vi "Data Logging.old.vi"(8 "error in (no error)":errorcluster, 11 "stop?":bool) -> (0 "error out":errorcluster)   [LabVIEW 2011]
uses:
  <vilib>/Utility/sysdir.llb/System Directory Type.ctl
  <vilib>/Platform/TimedLoop/XDataNode/timing_clust.ctl
  <vilib>/Platform/TimedLoop/XDataNode/nitl_modes.ctl
  <vilib>/Platform/TimedLoop/XDataNode/wakeup.ctl
  <vilib>/Platform/TimedLoop/XDataNode/XDataNode.xnode
  <vilib>/Platform/TimedLoop/XDataNode/XDNodeRunTimeDep.lvlib
panel:
  out "Data Cluster":T1
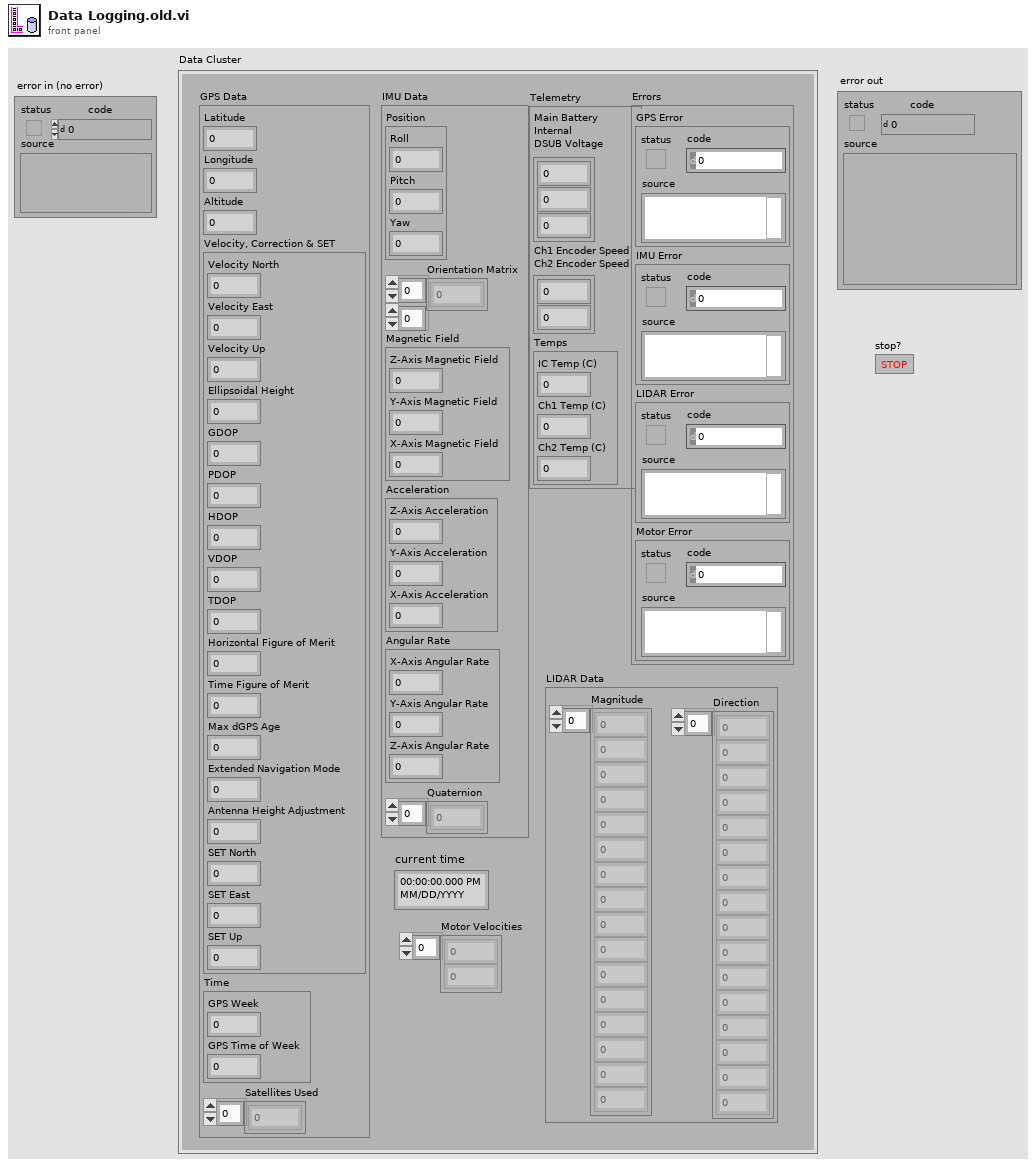
[diagram p1: front panel]
types:
  T1 = cluster{"GPS Data":cluster{"Latitude":dbl, "Longitude":dbl, "Altitude":dbl, "Velocity, Correction & SET":cluster{"Velocity North":dbl, "Velocity East":dbl, "Velocity Up":dbl, "Ellipsoidal Height":dbl, "GDOP":sgl, "PDOP":sgl, "HDOP":sgl, "VDOP":sgl, "TDOP":sgl, "Horizontal Figure of Merit":u8, "Time Figure of Merit":u8, "Max dGPS Age":sgl, "Extended Navigation Mode":u8, "Antenna Height Adjustment ":dbl, "SET North":i32, "SET East":i32, "SET Up":i32}, "Time":cluster{"GPS Week":u16, "GPS Time of Week":sgl}, "Satellites Used":i32[]}, "IMU Data":cluster{"Position":cluster{"Roll":dbl, "Pitch":dbl, "Yaw":dbl}, "Orientation Matrix":dbl[][], "Magnetic Field":cluster{"Z-Axis Magnetic Field":dbl, "Y-Axis Magnetic Field":dbl, "X-Axis Magnetic Field":dbl}, "Acceleration":cluster{"Z-Axis Acceleration":dbl, "Y-Axis Acceleration":dbl, "X-Axis Acceleration":dbl}, "Angular Rate":cluster{"X-Axis Angular Rate":dbl, "Y-Axis Angular Rate":dbl, "Z-Axis Angular Rate":dbl}, "Quaternion":dbl[]}, "Telemetry":cluster{"Main Battery\nInternal\nDSUB Voltage":cluster{sgl, sgl, sgl}, "Ch1 Encoder Speed\nCh2 Encoder Speed":cluster{i32, i32}, "Temps":cluster{"IC Temp (C)":i32, "Ch1 Temp (C)":i32, "Ch2 Temp (C)":i32}}, "Motor Velocities":dbl[], "Errors":cluster{"GPS Error ":errorcluster, "IMU Error":errorcluster, "LIDAR Error":errorcluster, "Motor Error":errorcluster}, "current time":timestamp, "LIDAR Data":cluster{"Magnitude":dbl[], "Direction":dbl[]}}
  T2 = enum16{"open", "replace", "create", "open or create", "replace or create", "replace or create with confirmation"}
  T3 = typedef "System Directory Type.ctl" = i32
  T4 = cluster{"GPS Error ":errorcluster, "IMU Error":errorcluster, "LIDAR Error":errorcluster, "Motor Error":errorcluster}
  T5 = typedef "XDNodeRunTimeDep.lvlib/timing_clust.ctl" = cluster{"Expected End [f-1]":u64, "Actual End [f-1]":u64, "Finished Late? [f-1]":bool, "Expected End [i-1]":u64, "Actual End [i-1]":u64, "Finished Late? [i-1]":bool, "Expected Start [i]":u64, "Actual Start [i]":u64, "Expected Start [f]":u64, "Actual Start [f]":u64, "Source Name":string, "Structure Name":string, "Period":i64, "Deadline":i64, "Offset":i64, "Start":i64, "Priority":i32, "Timeout":i32, "Mode":T6, "Wakeup Reason":T7, "Error":errorcluster, "Source Type":string, "Secondary Source Type":string, "Global End Time":u64, "Global Start Time":u64, "Frame Duration":u64, "Iteration Duration":u64, "Assigned CPU":i32, "I/O Scan Engine Mode":u32}
  T6 = typedef "XDNodeRunTimeDep.lvlib/nitl_modes.ctl" = enum32{"No Change", "Process missed periods, maintain original phase", "Discard missed periods, maintain original phase", "Process missed periods, ignore original phase", "Discard missed periods, ignore original phase"}
  T7 = typedef "XDNodeRunTimeDep.lvlib/wakeup.ctl" = enum32{"Normal", "Aborted", "Asynchronous wakeup", "Timing source error", "Timed loop error", "Timeout"}
  T8 = cluster{"Main Battery\nInternal\nDSUB Voltage":cluster{sgl, sgl, sgl}, "Ch1 Encoder Speed\nCh2 Encoder Speed":cluster{i32, i32}, "Temps":cluster{"IC Temp (C)":i32, "Ch1 Temp (C)":i32, "Ch2 Temp (C)":i32}}
  T9 = cluster{"Latitude":dbl, "Longitude":dbl, "Altitude":dbl, "Velocity, Correction & SET":cluster{"Velocity North":dbl, "Velocity East":dbl, "Velocity Up":dbl, "Ellipsoidal Height":dbl, "GDOP":sgl, "PDOP":sgl, "HDOP":sgl, "VDOP":sgl, "TDOP":sgl, "Horizontal Figure of Merit":u8, "Time Figure of Merit":u8, "Max dGPS Age":sgl, "Extended Navigation Mode":u8, "Antenna Height Adjustment ":dbl, "SET North":i32, "SET East":i32, "SET Up":i32}, "Time":cluster{"GPS Week":u16, "GPS Time of Week":sgl}, "Satellites Used":i32[]}
  T10 = cluster{"Position":cluster{"Roll":dbl, "Pitch":dbl, "Yaw":dbl}, "Orientation Matrix":dbl[][], "Magnetic Field":cluster{"Z-Axis Magnetic Field":dbl, "Y-Axis Magnetic Field":dbl, "X-Axis Magnetic Field":dbl}, "Acceleration":cluster{"Z-Axis Acceleration":dbl, "Y-Axis Acceleration":dbl, "X-Axis Acceleration":dbl}, "Angular Rate":cluster{"X-Axis Angular Rate":dbl, "Y-Axis Angular Rate":dbl, "Z-Axis Angular Rate":dbl}, "Quaternion":dbl[]}
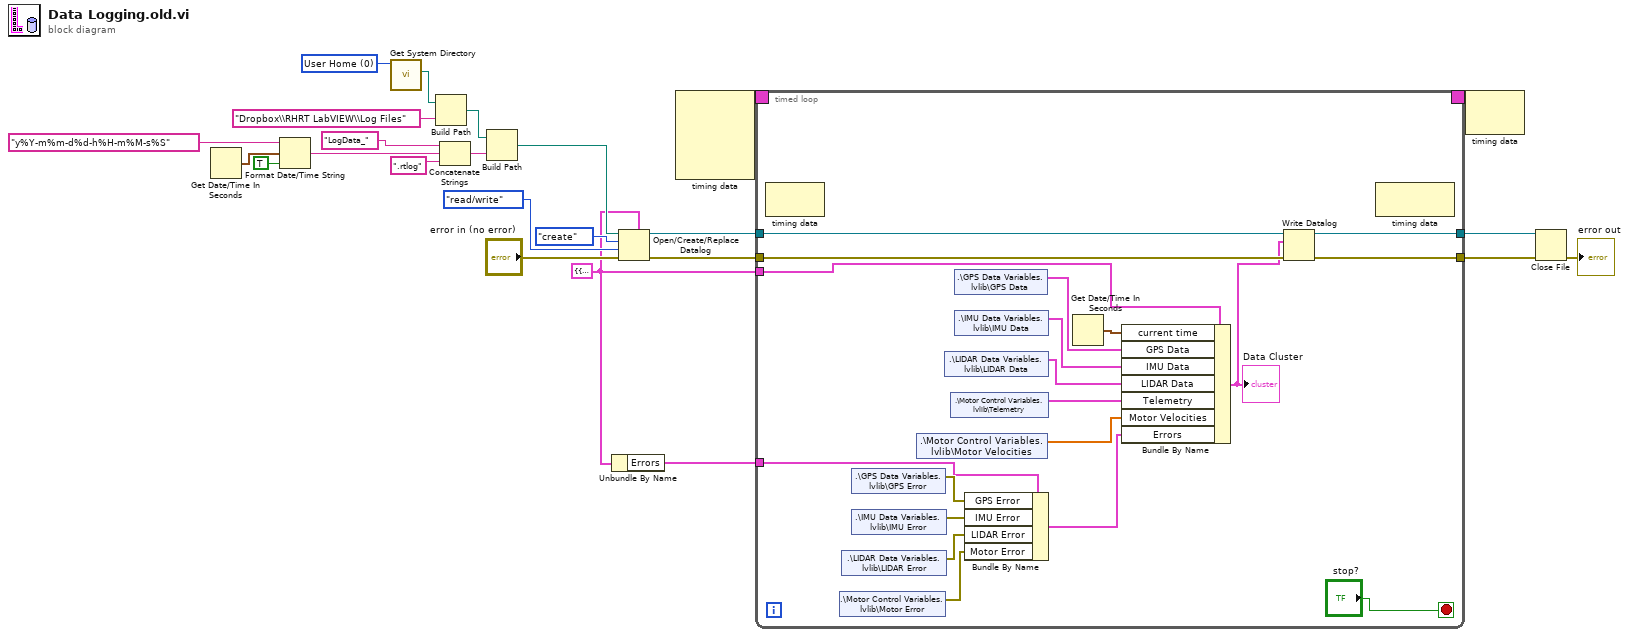
[diagram p0: block diagram]
diagram:
  w1 = T1 {"GPS Data"={"Latitude"=0.0, "Longitude"=0.0, "Altitude"=0.0, "Velocity, Correction & SET"={"Velocity North"=0.0, "Velocity East"=0.0, "Velocity Up"=0.0, "Ellipsoidal Height"=0.0, "GDOP"=0.0, "PDOP"=0.0, "HDOP"=0.0, "VDOP"=0.0, "TDOP"=0.0, "Horizontal Figure of Merit"=0, "Time Figure of Merit"=0, "Max dGPS Age"=0.0, "Extended Navigation Mode"=0, "Antenna Height Adjustment "=0.0, "SET North"=0, "SET East"=0, "SET Up"=0}, "Time"={"GPS Week"=0, "GPS Time of Week"=0.0}, "Satellites Used"=[]}, "IMU Data"={"Position"={"Roll"=0.0, "Pitch"=0.0, "Yaw"=0.0}, "Orientation Matrix"=[], "Magnetic Field"={"Z-Axis Magnetic Field"=0.0, "Y-Axis Magnetic Field"=0.0, "X-Axis Magnetic Field"=0.0}, "Acceleration"={"Z-Axis Acceleration"=0.0, "Y-Axis Acceleration"=0.0, "X-Axis Acceleration"=0.0}, "Angular Rate"={"X-Axis Angular Rate"=0.0, "Y-Axis Angular Rate"=0.0, "Z-Axis Angular Rate"=0.0}, "Quaternion"=[]}, "Telemetry"={"Main Battery\nInternal\nDSUB Voltage"={0.0, 0.0, 0.0}, "Ch1 Encoder Speed\nCh2 Encoder Speed"={0, 0}, "Temps"={"IC Temp (C)"=0, "Ch1 Temp (C)"=0, "Ch2 Temp (C)"=0}}, "Motor Velocities"=[], "Errors"={"GPS Error "={"status"=FALSE, "code"=0, "source"=""}, "IMU Error"={"status"=FALSE, "code"=0, "source"=""}, "LIDAR Error"={"status"=FALSE, "code"=0, "source"=""}, "Motor Error"={"status"=FALSE, "code"=0, "source"=""}}, "current time"=timestamp(0 s since 1904-01-01), "LIDAR Data"={"Magnitude"=[], "Direction"=[]}} ("Cluster")
  w9 = T3 0 items=["User Home"=0, "User Desktop"=1, "User Documents"=2, "User Application Data"=3, "User Preferences"=4, "User Temporary"=5, "Public Documents"=6, "Public Application Data"=7, "Public Preferences"=8, "Public Cache"=13, "System Core Libraries"=9, "System Installed Libraries"=10, "Application Files"=11, "Boot Volume Root"=12] ("system directory type")
  n1 = Get Date/Time In Seconds() -> (seconds since 1Jan1904=w15:timestamp)
  n2 = Format Date/Time String(time format string (%c)="y%Y-m%m-d%d-h%H-m%M-s%S", seconds (now)=w15, UTC format=TRUE) -> (date/time string=w13:string)
  n3 = call <vilib>:"Get System Directory.vi"("system directory type"=w9) -> ("system directory"=w7:path)  [unwired: 10 in]
  n4 = Build Path(base path=w7, name or relative path="Dropbox\\RHRT LabVIEW\\Log Files") -> (appended path=w8:path)
  n5 = Concatenate Strings("LogData_", w13, ".rtlog") -> (w10:string)
  n6 = Build Path(base path=w8, name or relative path=w10) -> (appended path=w5:path)
  n7 = Unbundle By Name(w1) -> ("Errors"=w4:T4)
  n8 = Open/Create/Replace Datalog(5:w1, 8:"error in (no error)", 9:enum16{"read/write", "read-only", "write-only"}."read/write" ("access (0:read/write)"), 10:T2."create" ("operation (0:open)"), 11:w5) -> (0:w21:errorcluster, 3:w20:refnum<k1>)  [unwired: 1 in, 1 out]
  n9 = node-c288() -> (w24:T5)  [unwired: 4 in]
  n10 = timed-loop {
    timing: w24 -> [_]
    timing-out: [_] -> w23
    tunnel: w1 -> [w38]
    tunnel: w21 -> [w37]
    tunnel: w20 -> [w36]
    tunnel: [w35] -> w19
    tunnel: [w34] -> w18
    tunnel: w4 -> [w29]
    stop <- "stop?" stop-if-true
    n11 = node-c288() -> ()  [unwired: 1 in, 1 out]
    n12 = shared-variable ".\\Motor Control Variables.lvlib\\Motor Error"() -> (w33:errorcluster)  [unwired: 1 in, 1 out]
    n13 = shared-variable ".\\LIDAR Data Variables.lvlib\\LIDAR Error"() -> (w32:errorcluster)  [unwired: 1 in, 1 out]
    n14 = shared-variable ".\\GPS Data Variables.lvlib\\GPS Error"() -> (w30:errorcluster)  [unwired: 1 in, 1 out]
    n15 = shared-variable ".\\IMU Data Variables.lvlib\\IMU Error"() -> (w31:errorcluster)  [unwired: 1 in, 1 out]
    n16 = shared-variable ".\\Motor Control Variables.lvlib\\Motor Velocities"() -> (w39:dbl[])  [unwired: 1 in, 1 out]
    n17 = shared-variable ".\\LIDAR Data Variables.lvlib\\LIDAR Data"() -> (w41:cluster{"Magnitude":dbl[], "Direction":dbl[]})  [unwired: 1 in, 1 out]
    n18 = shared-variable ".\\Motor Control Variables.lvlib\\Telemetry"() -> (w40:T8)  [unwired: 1 in, 1 out]
    n19 = shared-variable ".\\GPS Data Variables.lvlib\\GPS Data"() -> (w43:T9)  [unwired: 1 in, 1 out]
    n20 = shared-variable ".\\IMU Data Variables.lvlib\\IMU Data"() -> (w42:T10)  [unwired: 1 in, 1 out]
    n21 = Bundle By Name(cluster=w29, "GPS Error"=w30, "IMU Error"=w31, "LIDAR Error"=w32, "Motor Error"=w33) -> (w26:T4)
    n22 = Get Date/Time In Seconds() -> (seconds since 1Jan1904=w27:timestamp)
    n23 = Bundle By Name(cluster=w38, "current time"=w27, "GPS Data"=w43, "IMU Data"=w42, "LIDAR Data"=w41, "Telemetry"=w40, "Motor Velocities"=w39, "Errors"=w26) -> (w25:T1)
    "Data Cluster" <- w25
    n24 = Write Datalog(4:w37, 6:w25, 7:w36) -> (0:w35:errorcluster, 3:w34:refnum<k1>)
    n25 = node-c288() -> ()  [unwired: 1 in, 1 out]
  }
  n26 = node-c288(w23) -> ()  [unwired: 1 out]
  n27 = Close File(refnum=w18, error in=w19) -> (error out=→"error out":errorcluster)  [unwired: 1 out]
